vi "Create Instance Impl.vi"(8 "error in (no error)":errorcluster, 10 "Fluidics Configuration":T1={"Serial Port"="COM3", "Device Type"=enum."Disabled"}, 11 "Autosampler in":refnum<class "Alltesta Autosampler.lvclass">) -> (0 "error out":errorcluster, 3 "Autosampler out":refnum<class "Alltesta Autosampler.lvclass">)   [LabVIEW 2023, in "Alltesta Autosampler.lvlib" / "Alltesta Autosampler.lvclass"]
uses:
  Alltesta Autosampler.lvclass
  Alltesta Autosampler.lvclass/Alltesta Autosampler.ctl
  Alltesta Autosampler.lvlib
  Autosampler/Autosampler Needle Position.ctl
  Autosampler/Autosampler.lvlib
  Resources/Type Defs/Autosampler Configuration.ctl
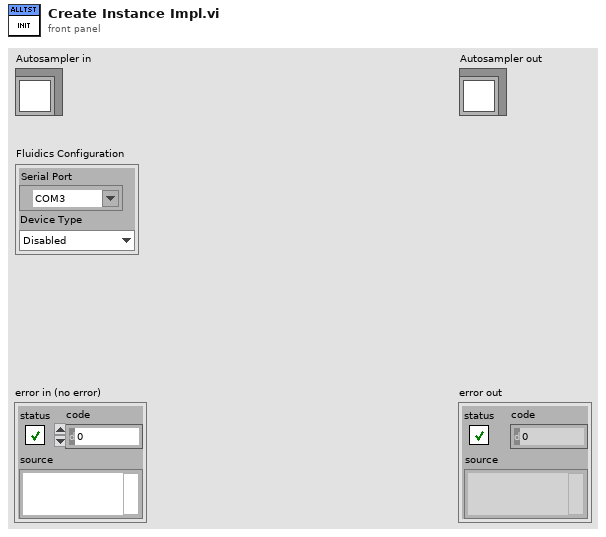
[diagram p1: front panel]
types:
  T1 = typedef "Autosampler Configuration.ctl" = cluster{"Serial Port":refnum<visa-resource-name>, "Device Type":enum16{"Disabled", "Simulate", "Alltesta"}}
  T2 = typedef "Autosampler.lvlib/Autosampler Needle Position.ctl" = enum16{"Down", "Up"}
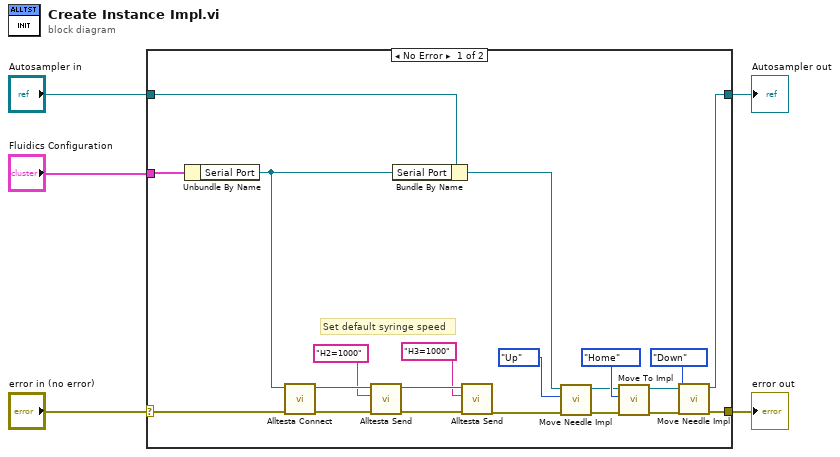
[diagram p0: block diagram]
diagram:
  n1 = case shown="No Error" "error in (no error)" {
    selector: "error in (no error)" -> [w24 w28]
    tunnel: [w10 w28] -> w4
    tunnel: "Autosampler in" -> [w26 w27]
    tunnel: [w8 w27] -> w2
    tunnel: "Fluidics Configuration" -> [w25 _]
    frame No Error {
      # "Set default syringe speed"
      n2 = Unbundle By Name(w25) -> ("Serial Port"=w23:refnum<visa-resource-name>)
      n3 = call "Alltesta Connect.vi"("error in (no error)"=w24, "VISA resource name"=w23) -> ("error out"=w22:errorcluster, "VISA resource name out"=w21:refnum<visa-resource-name>)  [unwired: 8 in]
      n4 = call "Alltesta Send.vi"("error in (no error)"=w22, "Command"="H2=1000", "Serial Port in"=w21) -> ("error out"=w20:errorcluster, "Serial Port out"=w19:refnum<visa-resource-name>)  [unwired: 5 in, 2 out]
      n5 = Bundle By Name(cluster=w26, "Serial Port"=w23) -> (w13:refnum<class "Alltesta Autosampler.lvclass">)
      n6 = call "Alltesta Send.vi"("error in (no error)"=w20, "Command"="H3=1000", "Serial Port in"=w19) -> ("error out"=w15:errorcluster)  [unwired: 5 in, 3 out]
      n7 = call-dynamic "Move Needle Impl.vi"("error in (no error)"=w15, "Needle Position"=Autosampler_Needle_Position."Up", "Alltesta Autosampler in"=w13) -> ("error out"=w14:errorcluster, "Alltesta Autosampler out"=w6:refnum<class "Alltesta Autosampler.lvclass">)  [unwired: 7 in]
      n8 = call-dynamic "Move To Impl.vi"("error in (no error)"=w14, "Area"=enum16{"Home", "Well", "Wash Port"}."Home", "Alltesta Autosampler in"=w6) -> ("error out"=w11:errorcluster, "Alltesta Autosampler out"=w9:refnum<class "Alltesta Autosampler.lvclass">)  [unwired: 7 in]
      n9 = call-dynamic "Move Needle Impl.vi"("error in (no error)"=w11, "Needle Position"=Autosampler_Needle_Position."Down", "Alltesta Autosampler in"=w9) -> ("error out"=w10:errorcluster, "Alltesta Autosampler out"=w8:refnum<class "Alltesta Autosampler.lvclass">)  [unwired: 7 in]
    }
    frame Error {
    }
  }
  "error out" <- w4
  "Autosampler out" <- w2
